vi "2dFloatArrayToString.vi"(1 "Value":sgl[][](array[numeric])) -> (0 "String":string)   [LabVIEW 2015]
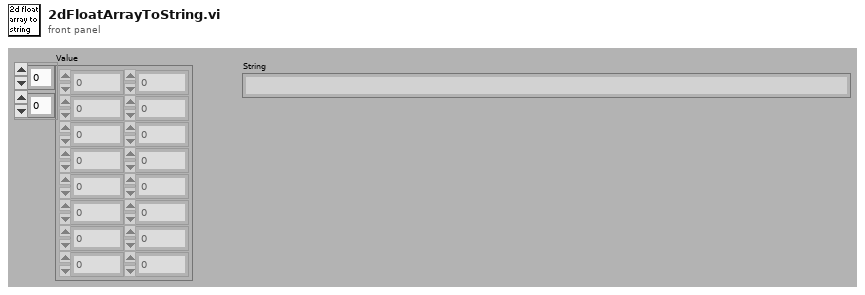
[diagram p1: front panel]
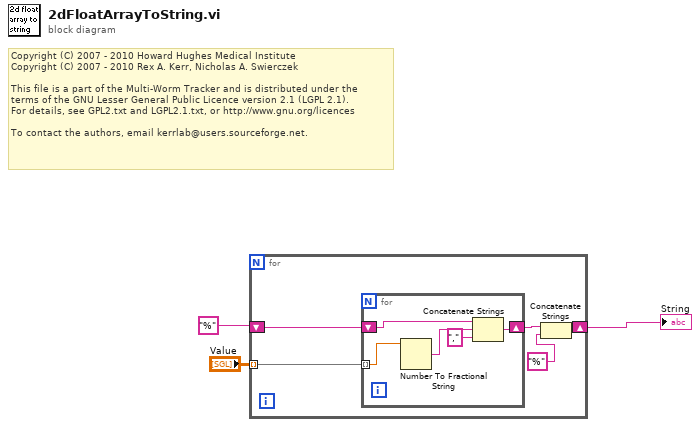
[diagram p0: block diagram]
diagram:
  # "Copyright (C) 2007 - 2010 Howard Hughes Medical Institute\nCopyright (C) 2007 - 2010 Rex A. Kerr, Nicholas A. Swierczek\n \nThis file is a part of the Multi-Worm Tracker and is distributed under the\nterms of the GNU Lesser General Public Licence version 2.1 (LGPL 2.1).\nFor details, see GPL2.txt and LGPL2.1.txt, or http://www.gnu.org/licences\n \nTo contact the authors, email kerrlab@users.sourceforge.net."
  n1 = for {
    tunnel: "Value" -> [w8] mode=indexing
    shift-right: [w5] -> w2
    shift-left: "%" -> [w4]
    n2 = for {
      tunnel: w8 -> [w12] mode=indexing
      shift-right: [w9] -> w7
      shift-left: w4 -> [w13]
      n3 = Number To Fractional String(number=w12) -> (F-format string=w11:string)  [unwired: 3 in]
      n4 = Concatenate Strings(w13, w11, "," ("string")) -> (w9:string)
    }
    n5 = Concatenate Strings(w7, "%") -> (w5:string)
  }
  "String" <- w2
